vi "Count_Ratio_Mov_Unmov-3.vi"(3 "error IN":errorcluster, 4 "[IN] Coordinates of Moving \nPoints (X,Y,dX,dY) Mixed and \nRecorded in Columns":dbl[][](array[numeric]), 5 "[IN] Arrays of Unmoving\nPoints (X,Y) recorded in \nColumns (after processing)":dbl[][](array[numeric])) -> (0 "error OUT":errorcluster, 2 "[OUT] Ratio of moving points in \n1 frame (column) to unmoving \npoints in the same frame (column)":i16[](array[numeric]))   [LabVIEW 2013]
panel:
  out "[OUT] Amount of moving \npoints recorded in columns":i16[](array[numeric])
  out "[OUT] Amount of unmoving \npoints recorded in columns":i16[](array[numeric])
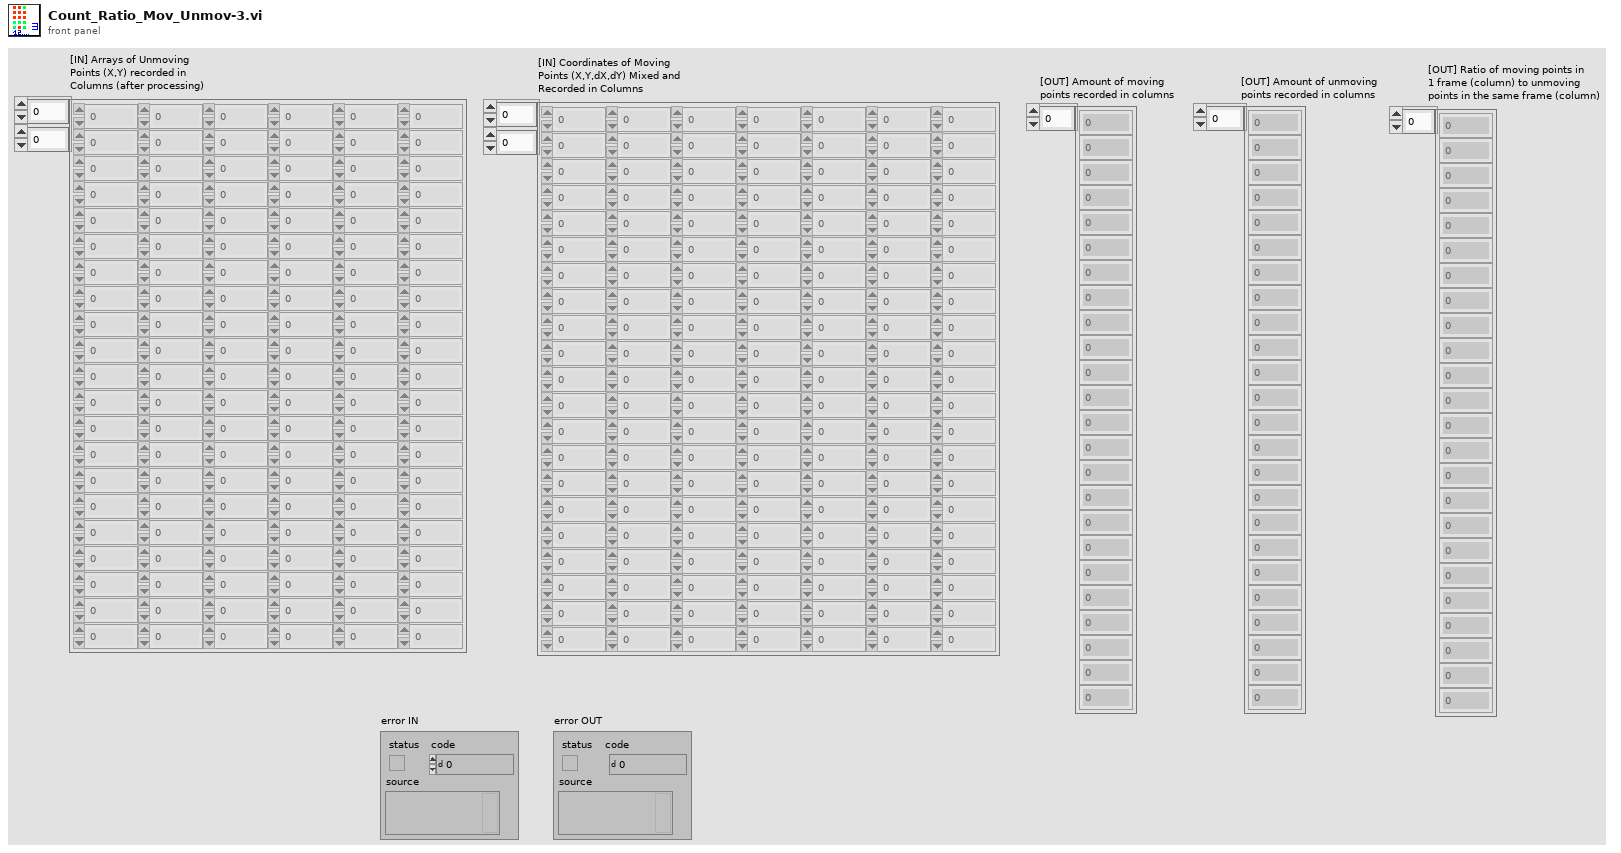
[diagram p1: front panel]
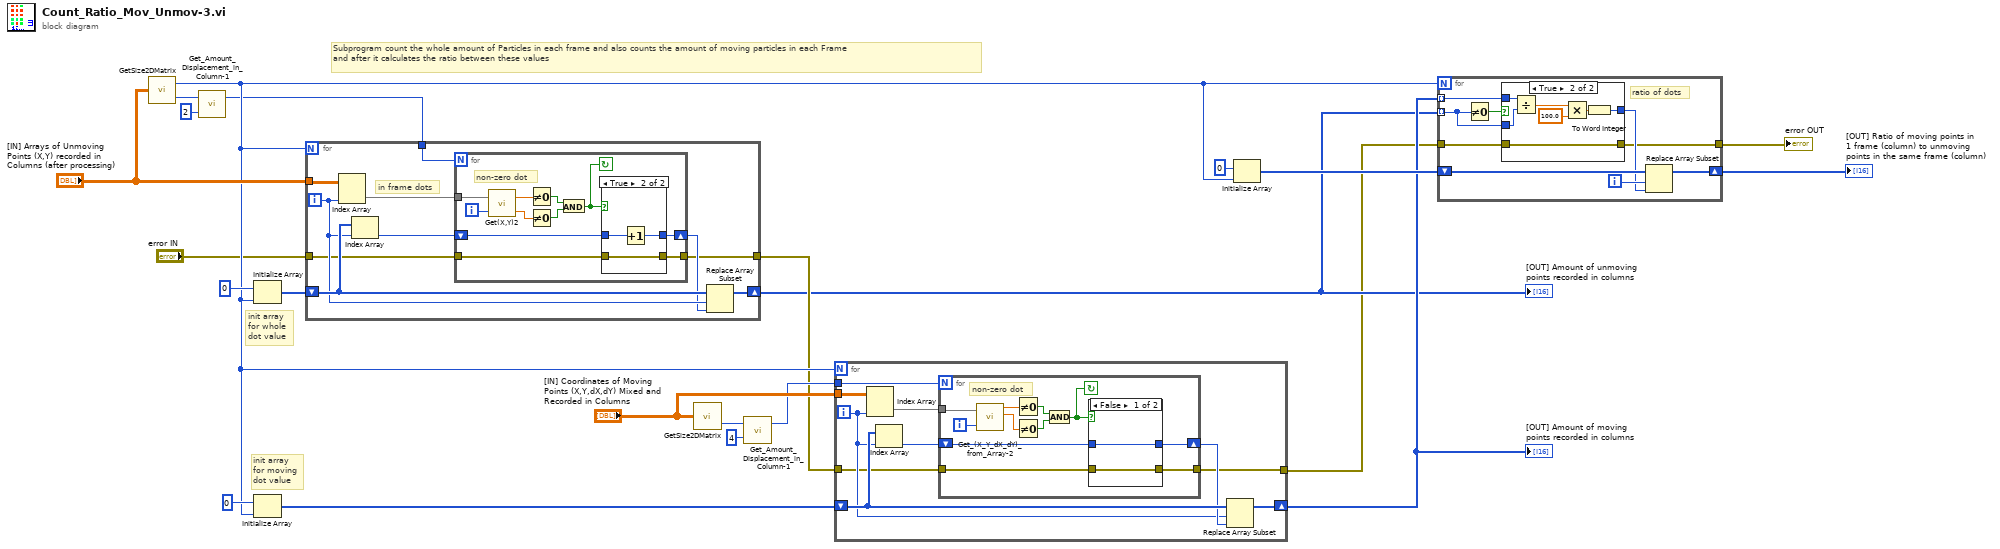
[diagram p0: block diagram]
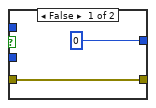
[diagram p2: hidden frame]
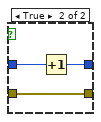
[diagram p3: hidden frame]
diagram:
  # "init array \nfor moving\ndot value"
  # "init array \nfor whole\ndot value"
  # "Subprogram count the whole amount of Particles in each frame and also counts the amount of moving particles in each Frame\nand after it calculates the ratio between these values"
  n1 = call "GetSize2DMatrix.vi"("Array IN (2D)"="[IN] Arrays of Unmoving\nPoints (X,Y) recorded in \nColumns (after processing)") -> ("# Cols"=w14:i32, "# Rows"=w10:i32)
  n2 = call "Get_Amount_Displacement_in_Column-1.vi"("multiplier"=2, "# Rows"=w10) -> ("Displ amount"=w9:i32)  [unwired: 1 out]
  n3 = Initialize Array(i16 0 ("element"), w14) -> (w21:i16[])
  n4 = Initialize Array(i16 0 ("element"), w14) -> (w19:i16[])
  n5 = for {
    N: w14 -> [_]
    shift-right: [w26] -> w3
    shift-left: w21 -> [w29]
    tunnel: "[IN] Arrays of Unmoving\nPoints (X,Y) recorded in \nColumns (after processing)" -> [w32]
    tunnel: w9 -> [w25]
    tunnel: "error IN" -> [w24]
    tunnel: [w23] -> w4
    i -> [w28]
    # "in frame dots"
    n6 = Index Array(array=w32, index (col)=w28) -> (element=w31:dbl[])  [unwired: 1 in]
    n7 = Index Array(array=w29, index=w28) -> (element=w30:i16)
    n8 = for {
      N: w25 -> [_]
      tunnel: w31 -> [w39]
      shift-right: [w40] -> w27
      shift-left: w30 -> [w41]
      tunnel: w24 -> [w34]
      tunnel: [w33] -> w23
      i -> [w38]
      stop <- w35 continue-if-true
      # "non-zero dot"
      n9 = call "Get(X,Y)2.vi"("[IN] index of (X,Y)"=w38, "[IN] Array coordi\nnates (X,Y) in Frame"=w39) -> ("[OUT] Y"=w36:dbl, "[OUT] X"=w37:dbl)
      n10 = Not Equal To 0?(x=w37) -> (x != 0?=w43:bool)
      n11 = Not Equal To 0?(x=w36) -> (x != 0?=w42:bool)
      n12 = And(x=w43, y=w42) -> (x .and. y?=w35:bool)
      n13 = case shown="True" w35 {
        tunnel: w41 -> [w45 w48]
        tunnel: [w45 w47] -> w40
        tunnel: w34 -> [w44 w46]
        tunnel: [w44 w46] -> w33
        frame False {
        }
        frame True {
          n14 = Increment(x=w48) -> (x+1=w47:i16)
        }
      }
    }
    n15 = Replace Array Subset(array=w29, new element=w27, index=w28) -> (w26:i16[])
  }
  "[OUT] Amount of unmoving \npoints recorded in columns" <- w3
  n16 = call "GetSize2DMatrix.vi"("Array IN (2D)"="[IN] Coordinates of Moving \nPoints (X,Y,dX,dY) Mixed and \nRecorded in Columns") -> ("# Rows"=w7:i32)  [unwired: 1 out]
  n17 = call "Get_Amount_Displacement_in_Column-1.vi"("multiplier"=4, "# Rows"=w7) -> ("Displ amount"=w6:i32)  [unwired: 1 out]
  n18 = for {
    N: w14 -> [_]
    shift-right: [w53] -> w13
    shift-left: w19 -> [w55]
    tunnel: "[IN] Coordinates of Moving \nPoints (X,Y,dX,dY) Mixed and \nRecorded in Columns" -> [w58]
    tunnel: w6 -> [w51]
    tunnel: w4 -> [w50]
    tunnel: [w49] -> w2
    i -> [w52]
    n19 = Index Array(array=w58, index (col)=w52) -> (element=w57:dbl[])  [unwired: 1 in]
    n20 = Index Array(array=w55, index=w52) -> (element=w56:i16)
    n21 = for {
      N: w51 -> [_]
      tunnel: w57 -> [w64]
      shift-right: [w67] -> w54
      shift-left: w56 -> [w65]
      tunnel: w50 -> [w60]
      tunnel: [w59] -> w49
      i -> [w63]
      stop <- w66 continue-if-true
      # "non-zero dot"
      n22 = call "Get_(X_Y_dX_dY)_from_Array-2.vi"("(X,Y,dX,dY)"=w64, "Index of Displacement"=w63) -> ("X"=w62:dbl, "Y"=w61:dbl)  [unwired: 2 out]
      n23 = Not Equal To 0?(x=w62) -> (x != 0?=w69:bool)
      n24 = Not Equal To 0?(x=w61) -> (x != 0?=w68:bool)
      n25 = And(x=w69, y=w68) -> (x .and. y?=w66:bool)
      n26 = case shown="False" w66 {
        tunnel: w65 -> [w71 w74]
        tunnel: [w71 w73] -> w67
        tunnel: w60 -> [w70 w72]
        tunnel: [w70 w72] -> w59
        frame False {
        }
        frame True {
          n27 = Increment(x=w74) -> (x+1=w73:i16)
        }
      }
    }
    n28 = Replace Array Subset(array=w55, new element=w54, index=w52) -> (w53:i16[])
  }
  "[OUT] Amount of moving \npoints recorded in columns" <- w13
  n29 = Initialize Array(i16 0 ("element"), w14) -> (w17:i16[])
  n30 = for {
    N: w14 -> [_]
    shift-right: [w79] -> w16
    shift-left: w17 -> [w82]
    tunnel: w3 -> [w77] mode=indexing
    tunnel: w13 -> [w83] mode=indexing
    tunnel: w2 -> [w76]
    tunnel: [w75] -> w1
    i -> [w81]
    # "ratio of dots"
    n31 = Not Equal To 0?(x=w77) -> (x != 0?=w78:bool)
    n32 = case shown="True" w78 {
      tunnel: w83 -> [_ w92]
      tunnel: [i16 0 w88] -> w80
      tunnel: w77 -> [_ w87]
      tunnel: w76 -> [w84 w86]
      tunnel: [w84 w86] -> w75
      frame False {
      }
      frame True {
        n33 = Divide(x=w92, y=w87) -> (x/y=w91:dbl)
        n34 = Multiply(x=w91, y=100.0) -> (x*y=w89:dbl)
        n35 = To Word Integer(number=w89) -> (16bit integer=w88:i16)
      }
    }
    n36 = Replace Array Subset(array=w82, new element=w80, index=w81) -> (w79:i16[])
  }
  "error OUT" <- w1
  "[OUT] Ratio of moving points in \n1 frame (column) to unmoving \npoints in the same frame (column)" <- w16
